vi "set_path_group.vi"(2 "error in (no error)":errorcluster, 3 "Path":path, 4 "Experiments_group.lvclass in":refnum<class "Experiments_group.lvclass">) -> (0 "error out":errorcluster, 1 "Experiments_group.lvclass out":refnum<class "Experiments_group.lvclass">)   [LabVIEW 2015, in "Experiments_group.lvclass"]
uses:
  Experiments_group.lvclass
  Experiments_group.lvclass/Experiments_group.ctl
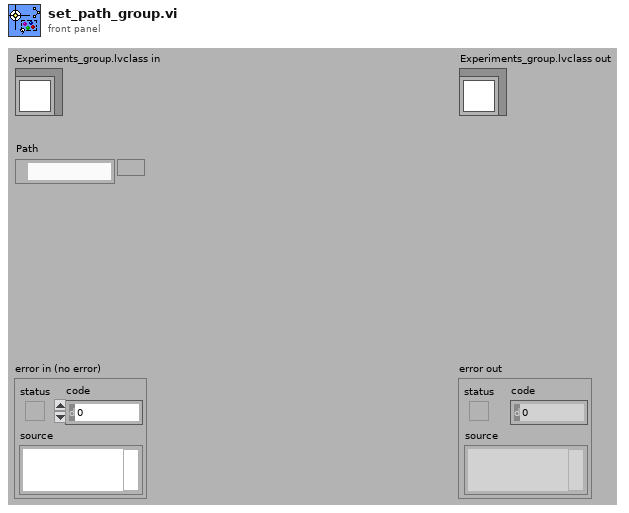
[diagram p1: front panel]
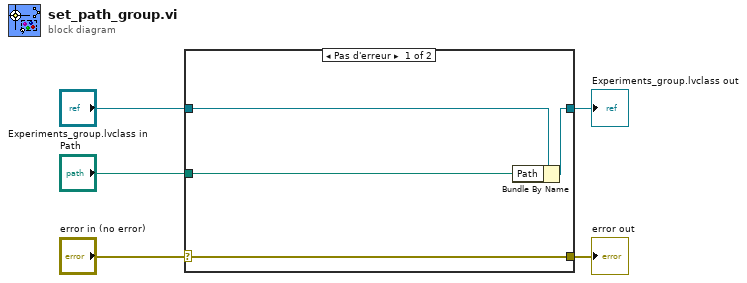
[diagram p0: block diagram]
diagram:
  n1 = case shown="Pas d'erreur" "error in (no error)" {
    selector: "error in (no error)" -> [w9 w10]
    tunnel: [w9 w10] -> w4
    tunnel: [w7 w11] -> w2
    tunnel: "Experiments_group.lvclass in" -> [w8 w11]
    tunnel: "Path" -> [w6 _]
    frame No Error {
      n2 = Bundle By Name(cluster=w8, "Path"=w6) -> (w7:refnum<class "Experiments_group.lvclass">)
    }
    frame Error {
    }
  }
  "error out" <- w4
  "Experiments_group.lvclass out" <- w2
